vi "Read Instruments.vi"(0 "Experiment in":refnum<class "Experiment.lvclass">) -> (12 "state":T1(ring), 13 "Analog_Input":refnum<class "Analog_Input.lvclass">, 14 "Experiment out":refnum<class "Experiment.lvclass">, 15 "ExperimentVariables.lvclass":refnum<class "ExperimentVariables.lvclass">, 16 "Camera":refnum<class "Camera.lvclass">, 17 "HSDIO":refnum<class "HSDIO.lvclass">, 18 "DAQmx_pulse_out":refnum<class "DAQmx_pulse_out.lvclass">, 19 "Analog_Output":refnum<class "Analog_Output.lvclass">)   [LabVIEW 2013, in "Experiment.lvclass"]
uses:
  Experiment.lvclass
  ExperimentVariables/ExperimentVariables.lvclass
  Camera/Camera.lvclass
  HSDIO/HSDIO.lvclass
  DAQmx_pulse_out/DAQmx_pulse_out.lvclass
  Analog_output/Analog_Output.lvclass
  Analog_Input/Analog_Input.lvclass
  Experiment.lvclass/Experiment.ctl
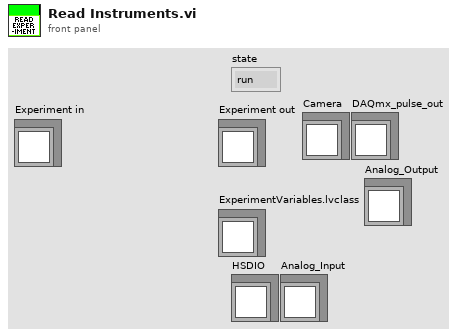
[diagram p1: front panel]
types:
  T1 = enum16{"run", "pause", "shutdown gracefully", "halt immediately"}
  T2 = typedef "states.ctl" = enum16{"run", "pause", "shutdown gracefully", "halt immediately", "waiting for connection", "waiting for command"}
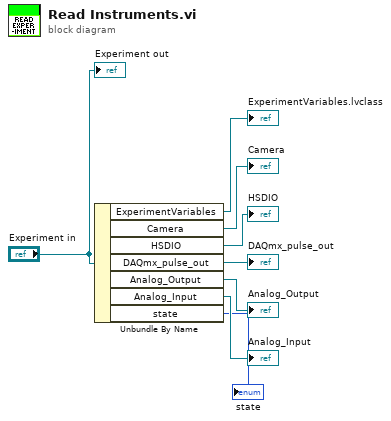
[diagram p0: block diagram]
diagram:
  n1 = Unbundle By Name("Experiment in") -> ("ExperimentVariables"=→"ExperimentVariables.lvclass":refnum<class "ExperimentVariables.lvclass">, "Camera"=→"Camera":refnum<class "Camera.lvclass">, "HSDIO"=→"HSDIO":refnum<class "HSDIO.lvclass">, "DAQmx_pulse_out"=→"DAQmx_pulse_out":refnum<class "DAQmx_pulse_out.lvclass">, "Analog_Output"=→"Analog_Output":refnum<class "Analog_Output.lvclass">, "Analog_Input"=→"Analog_Input":refnum<class "Analog_Input.lvclass">, "state"=→"state":T2)
  "Experiment out" <- "Experiment in"
